vi "name to card channel one-off.vi"   [LabVIEW 2018]
uses:
  channel_cluster.ctl
  <vilib>/Utility/file.llb/Write Delimited Spreadsheet (string).vi
types:
  T1 = typedef "channel_cluster.ctl" = cluster{"Channel Name":string, "Crate":i32, "Card Type":string, "Card":i32, "Channel":i32, "Status Icon":picture, "Vmon (V)":dbl, "Vset (V)":dbl, "Imon (A)":dbl, "Iset (A)":dbl, "Timestamp":string, "ON/OFF":bool, "Status":string, "Vswmax (V)":dbl, "Flag":bool, "Vfile (V)":dbl, "Error Logged":bool[]}
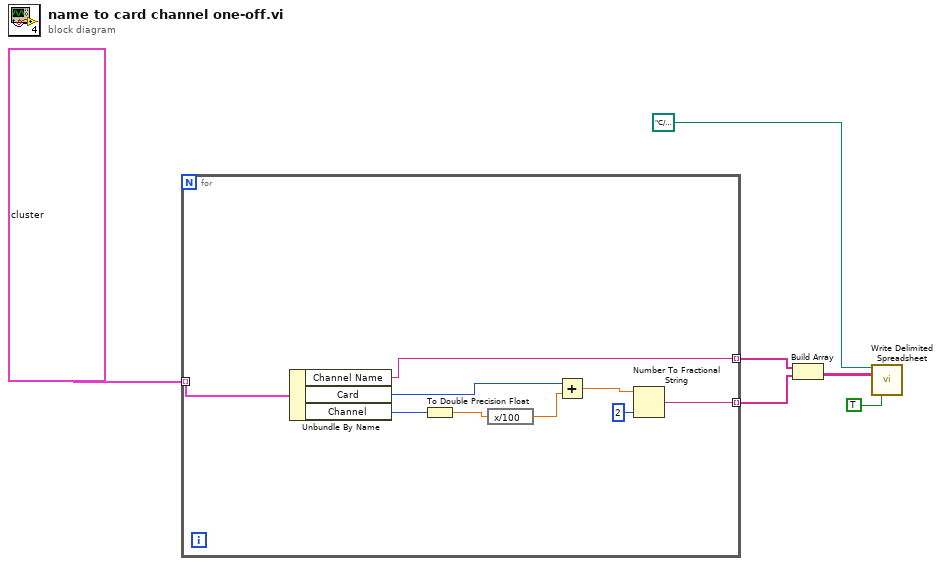
[diagram p0: block diagram]
diagram:
  n1 = for {
    tunnel: T1[] data[141878B] ("Channel Array") -> [w15] mode=indexing
    tunnel: [w8] -> w6 mode=indexing
    tunnel: [w7] -> w5 mode=indexing
    n2 = Unbundle By Name(w15) -> ("Channel Name"=w8:string, "Card"=w11:i32, "Channel"=w14:i32)
    n3 = To Double Precision Float(number=w14) -> (double precision float=w13:dbl)
    n4 = expression code="x/100"(w13) -> (w12:dbl)
    n5 = Add(x=w11, y=w12) -> (x+y=w10:dbl)
    n6 = Number To Fractional String(number=w10, precision (6)=i16 2) -> (F-format string=w7:string)  [unwired: 2 in]
  }
  n7 = Build Array(w6, w5) -> (w4:string[][])
  n8 = call-poly <vilib>:"Write Delimited Spreadsheet.vi"("file path (dialog if empty)"=path "C:/Users/ANNIE/Documents/names.txt", "2D data"=w4, "transpose? (no:F)"=TRUE ("transpose? (F)")) -> ()  [unwired: 11 in, 2 out]
